vi "subvi_Read_tdms.vi"(8 "Error In":errorcluster caption="에러 입력", 9 "카운트(-1: 전체)":i64, 10 "오프셋(0)":i64, 11 "selected path":path) -> (0 "Error Out":errorcluster caption="에러 출력", 1 "data":waveform(dbl)[](array[waveform]))   [LabVIEW 2016]
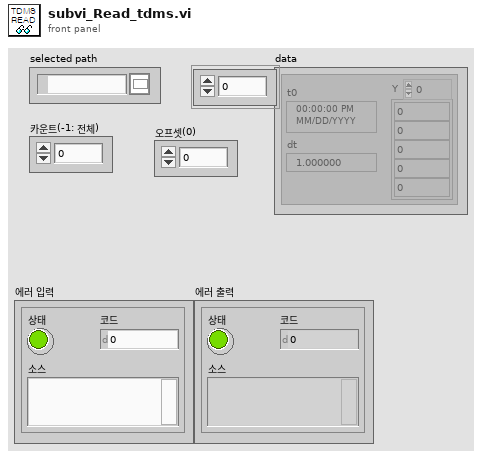
[diagram p1: front panel]
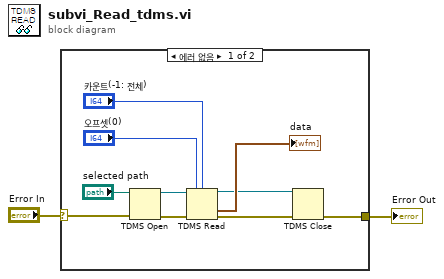
[diagram p0: block diagram]
diagram:
  n1 = case shown="에러 없음" "Error In" {
    selector: "Error In" -> [w8 w13]
    tunnel: [w7 w13] -> w1
    frame No Error {
      n2 = TDMS Open(8:w8, 11:"selected path") -> (0:w3:errorcluster, 3:w5:refnum<k34>)  [unwired: 5 in]
      n3 = TDMS Read(0:w5, 1:"오프셋(0)", 2:"카운트(-1: 전체)", 11:w3) -> (4:w6:refnum<k34>, 10:→"data":waveform(dbl)[], 15:w4:errorcluster)  [unwired: 4 in, 3 out]
      n4 = TDMS Close(8:w4, 11:w6) -> (0:w7:errorcluster)  [unwired: 1 out]
    }
    frame Error {
    }
  }
  "Error Out" <- w1
